vi "Priority.vi"(8 "error in (no error)":errorcluster, 11 "Session Cleanup Handler in":refnum<class "Session Cleanup Handler.lvclass">) -> (0 "error out":errorcluster, 2 "Priority":u16, 3 "Session Cleanup Handler out":refnum<class "Session Cleanup Handler.lvclass">)   [LabVIEW 2020, in "HTTP Server.lvlib" / "Session Cleanup Handler.lvclass"]
uses:
  Session Cleanup Handler.lvclass
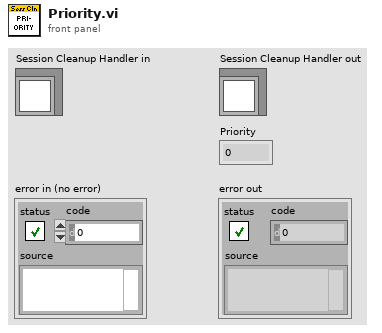
[diagram p1: front panel]
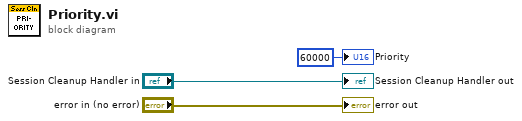
[diagram p0: block diagram]
diagram:
  "error out" <- "error in (no error)"
  "Session Cleanup Handler out" <- "Session Cleanup Handler in"
  "Priority" <- u16 60000 ("Priority")
